vi "OScStatus-com-exec.vi"(8 "error in (no error)":errorcluster, 10 "WCM_state":bool, 11 "Oscilloscope in":refnum<class "Oscilloscope.lvclass">) -> (0 "error out":errorcluster, 3 "Oscilloscope out":refnum<class "Oscilloscope.lvclass">)   [LabVIEW 2015, in "Oscilloscope.lvclass"]
uses:
  Oscilloscope.lvclass
  dependecies/ControlsVIs/Clusters-def/Message types.ctl
  dependecies/ControlsVIs/Clusters-def/SERVER-Commands.ctl
  dependecies/ControlsVIs/Clusters-def/OSc-Reply-Connect-Client.ctl
  GeneralFunctionality/GeneralFunctionality.lvclass/GeneralFunctionality.ctl
  Control/Control-Server/Control-Server.lvclass
  Message/Message.lvclass
  GeneralFunctionality/GeneralFunctionality.lvclass
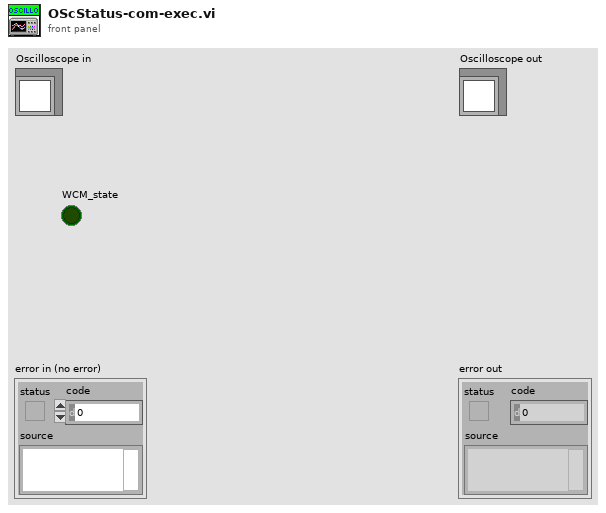
[diagram p1: front panel]
types:
  T1 = typedef "Oscilloscope.lvclass/OSc-Reply-Connect-Client.ctl" = cluster{"on/off":bool, "WCM_state":bool, "error":errorcluster}
  T2 = typedef "Control-Server.lvclass/SERVER-Commands.ctl" = string
  T3 = typedef "Message types.ctl" = string
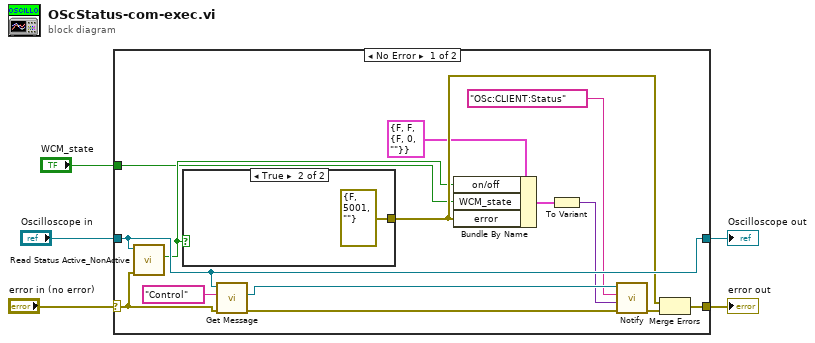
[diagram p0: block diagram]
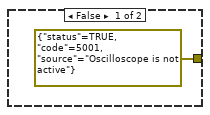
[diagram p2: hidden frame]
diagram:
  n1 = case shown="No Error" "error in (no error)" {
    selector: "error in (no error)" -> [w9 w23]
    tunnel: [w16 w23] -> w3
    tunnel: [w14 w22] -> w2
    tunnel: "Oscilloscope in" -> [w14 w22]
    tunnel: "WCM_state" -> [w6 _]
    frame No Error {
      n2 = call "Read Status Active_NonActive.vi"("error in (no error)"=w9, "GeneralFunctionality in"=w14) -> ("Status Active/NonActive"=w7:bool)  [unwired: 7 in, 2 out]
      n3 = case shown="True" w7 {
        tunnel: [errorcluster {"status"=TRUE, "code"=5001, "source"="Oscilloscope is not active"} ("error") errorcluster {"status"=FALSE, "code"=5001, "source"=""} ("error")] -> w10
        frame False {
        }
        frame True {
        }
      }
      n4 = call "Get Message.vi"("error in (no error)"=w9, "Message type"=T3 "Control", "GeneralFunctionality en entrée"=w14) -> ("error out"=w15:errorcluster, "Message.lvclass"=w19:refnum<class "Message.lvclass">)  [unwired: 6 in, 1 out]
      n5 = Bundle By Name(cluster=T1 {"on/off"=FALSE, "WCM_state"=FALSE, "error"={"status"=FALSE, "code"=0, "source"=""}} ("output cluster"), "on/off"=w7, "WCM_state"=w6, "error"=w10) -> (w13:T1)
      n6 = To Variant(anything=w13) -> (Variant=w12:variant)
      n7 = call "Notify.vi"("error in (no error)"=w15, "Data"=w12, "command"=T2 "OSc:CLIENT:Status" ("Commands"), "Message en entrée"=w19) -> ("error out"=w17:errorcluster)  [unwired: 6 in, 1 out]
      n8 = Merge Errors(w10, w17) -> (w16:errorcluster)
    }
    frame Error {
    }
  }
  "error out" <- w3
  "Oscilloscope out" <- w2
